vi "Add and Update Devicetype Variable in DB.vi"(8 "error in":errorcluster, 9 "Dont Set variables list":string[](array[string]), 10 "Devicetype variable\nCluster Data":string[][](array[string]), 11 "Device Name":string) -> (0 "error out":errorcluster, 3 "Devicetype \nvariable DB data":string[][](array[string]))   [LabVIEW 2020]
doc: "Thsis vi Update and Add Devicetype Variable in database by analysing Setings Cluster Data\nInput:\n1. Settins Cluster Data\n2. DeviceName\n3.Error In\n\nOutput:\n1. Devicetype Variable list\n2. Error out"
uses:
  Preset Query Enum.ctl
  source/Device Drivers/BaseDriver/BaseDriver.lvclass
panel:
  out "subarray":string[](array[string])
  out "Array":string[][](array[string])
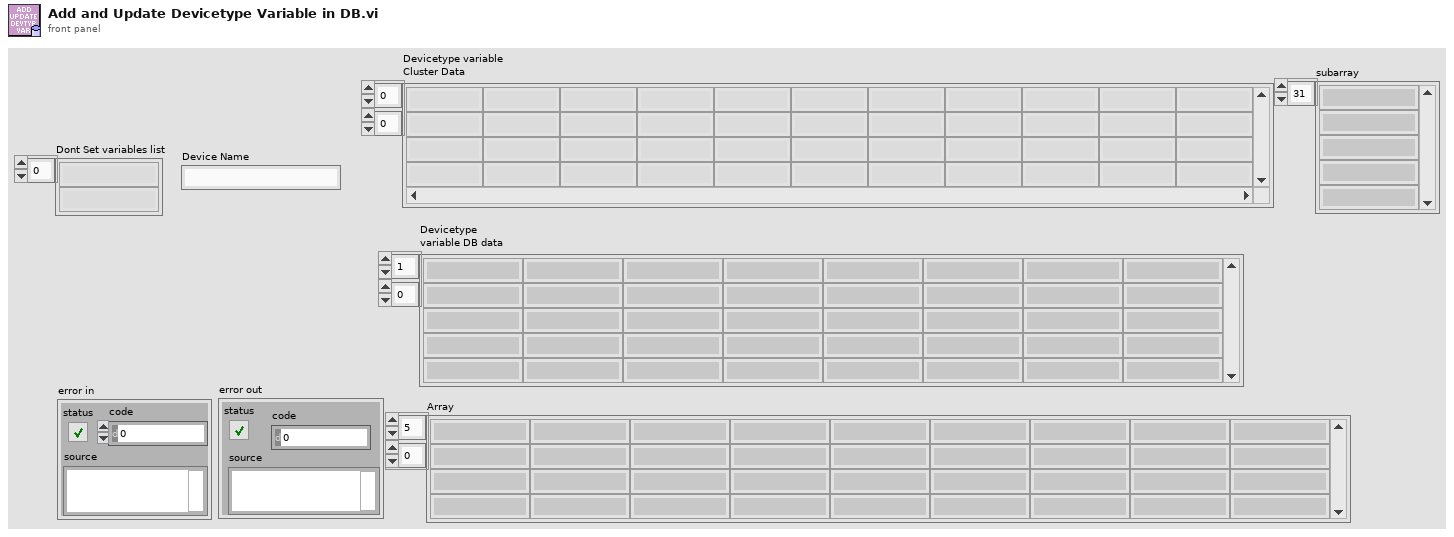
[diagram p1: front panel]
types:
  T1 = typedef "Preset Query Enum.ctl" = enum16{"Get Locations", "Get all IPs and MACs", "Get classes", "Get expt variables to set at scanstart for particular device", "Get expt devices and variables with start values", "Get expt devices and variables (with data to get)", "Get expt devices with data to get", "Get Expt devices and GUIs", "Get all devices basic properties", "Get Virtual Devices Core Info", "Get Expt names", "Get experiment basic properties", "Get experiment alarm variables", "Get MC Ports", "Get device network comm port", "Get devicetype lvclass path", "Get basic device properties", "Get Init Order", "Get all setable variables of a device", "Get device variable aliases", "Get force values of all settable variables", "Get all variables of a devicetype", "Get all variables of a device", "Get plotter details", "Get Saved Scans", "Get Scan Info", "GetGeneralGUIs", "Get expt for plotter", "Get plotter IDs from expt", "Get all devices", "Get all Virtual Devices", "Get all aliases", "Get variable and device info for Virtual Device", "GetItemLocatorIP", "Get IPs for GUIs", "Get DeviceType from Device", "GetLocalPortRange", "GetDevicePresetVariables", "Get Device Configuration", "GetAllPresetNames", "GetAllConfigurationNames", "GetPresetDeviceNames"}
  T2 = typedef "mysql_authentication.ctl" = cluster{"User":string, "Password":string, "Database":string}
  T3 = cluster{"Port":u16, "IP Address":string, "Authentication":T2}
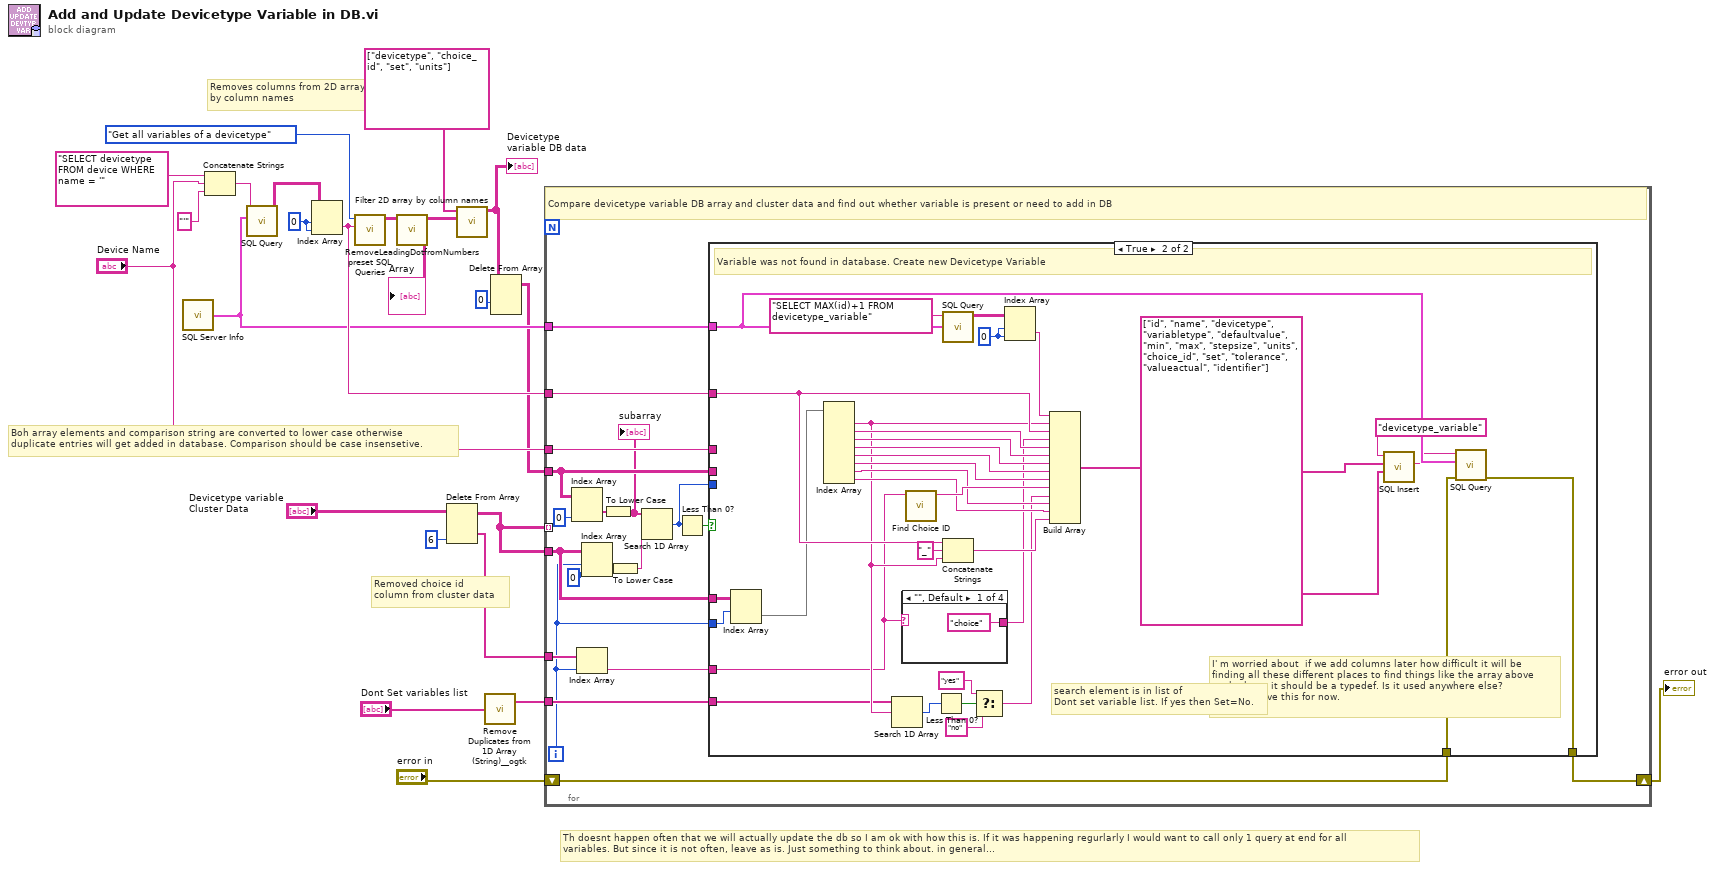
[diagram p0: block diagram]
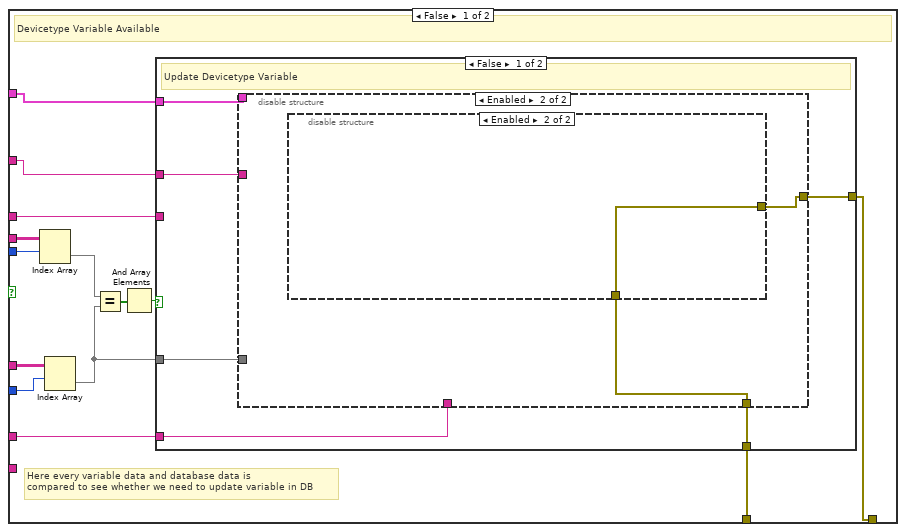
[diagram p2: hidden frame]
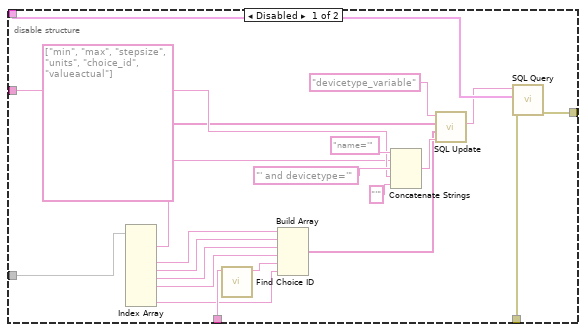
[diagram p3: hidden frame]
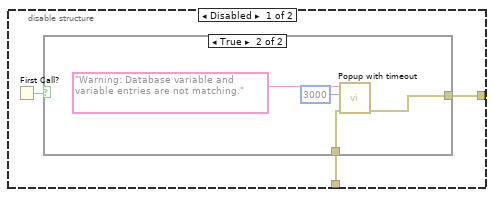
[diagram p4: hidden frame]
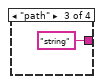
[diagram p8: hidden frame]
diagram:
  w15 = 0 ("disabled index (col)")
  # "Boh array elements and comparison string are converted to lower case otherwise \nduplicate entries will get added in database. Comparison should be case insensetive."
  # "Removed choice id\ncolumn from cluster data"
  # "Removes columns from 2D array\nby column names"
  # "Th doesnt happen often that we will actually update the db so I am ok with how this is. If it was happening regurlarly I would want to call only 1 query at end for all\nvariables. But since it is not often, leave as is. Just something to think about. in general..."
  n1 = call "SQL Server Info.vi"() -> ("SQL Server Info"=w14:T3)
  n2 = Concatenate Strings("SELECT devicetype FROM device WHERE name = '" ("Query"), "Device Name", "'" ("string")) -> (w13:string)
  n3 = call "SQL Query.vi"("SQL Server Info"=w14, "Query"=w13) -> ("data"=w16:string[][])  [unwired: 8 in, 1 out]
  n4 = Index Array(array=w16, index (row)=w15, index (col)=w15) -> (element=w20:string)
  n5 = call "preset SQL Queries.vi"("Device/Devicetype name\n/Plotter.id/ScanName#"=w20, "Preset Query"=Preset_Query_Enum."Get all variables of a devicetype") -> ("data"=w18:string[][])  [unwired: 7 in, 2 out]
  n6 = call "RemoveLeadingDotfromNumbers.vi"("data"=w18) -> ("Array"=w5:string[][])  [unwired: 10 in]
  "Array" <- w5
  n7 = Delete From Array(array="Devicetype variable\nCluster Data", index (col)=6 ("disabled index (col)")) -> (deleted portion=w22:string[], array with subset deleted=w23:string[][])  [unwired: 2 in]
  n8 = call "Filter 2D array by column names.vi"("Array in"=w5, "Array 3"=string[] ["devicetype", "choice_id", "set", "units"]) -> ("Array out"=w4:string[][])  [unwired: 9 in]
  "Devicetype \nvariable DB data" <- w4
  n9 = call "Remove Duplicates from 1D Array (String)__ogtk.vi"("Input Array"="Dont Set variables list") -> ("Output Array"=w7:string[])  [unwired: 1 out]
  n10 = Delete From Array(array=w4, index (row)=0) -> (array with subset deleted=w2:string[][])  [unwired: 2 in, 1 out]
  n11 = for {
    tunnel: w23 -> [w39]
    tunnel: w2 -> [w33]
    tunnel: w23 -> [_] mode=indexing
    tunnel: w14 -> [w38]
    tunnel: w20 -> [w34]
    shift-right: [w37] -> w9
    shift-left: "error in" -> [w36]
    tunnel: "Device Name" -> [w35]
    tunnel: w22 -> [w31]
    tunnel: w7 -> [w32]
    i -> [w30]
    # "Compare devicetype variable DB array and cluster data and find out whether variable is present or need to add in DB"
    n12 = Index Array(array=w33, index (col)=0) -> (element=w26:string[])  [unwired: 1 in]
    n13 = Index Array(array=w31, index=w30) -> (element=w29:string)
    n14 = Index Array(array=w39, index (row)=w30, index (col)=0 ("disabled index (col)")) -> (element=w27:string)
    n15 = To Lower Case(string=w26) -> (all lower case string=w25:string[])
    "subarray" <- w25
    n16 = To Lower Case(string=w27) -> (all lower case string=w24:string)
    n17 = Search 1D Array(1D array=w25, element=w24) -> (index of element=w28:i32)  [unwired: 1 in]
    n18 = Less Than 0?(x=w28) -> (x < 0?=w40:bool)
    n19 = case shown="True" w40 {
      tunnel: w33 -> [w56 _]
      tunnel: w39 -> [w55 w125]
      tunnel: w30 -> [w54 w124]
      tunnel: w38 -> [w48 w111]
      tunnel: w34 -> [w49 w116]
      tunnel: w36 -> [w47 w113]
      tunnel: [w46 w112] -> w37
      tunnel: w35 -> [w45 _]
      tunnel: w29 -> [w44 w99]
      tunnel: w32 -> [_ w106]
      tunnel: w28 -> [w43 _]
      frame False {
        # "Here every variable data and database data is \ncompared to see whether we need to update variable in DB"
        # "Devicetype Variable Available"
        n20 = Index Array(array=w56, index (row)=w43) -> (element=w52:string[])  [unwired: 1 in]
        n21 = Index Array(array=w55, index (row)=w54) -> (element=w50:string[])  [unwired: 1 in]
        n22 = Equal?(x=w52, y=w50) -> (x = y?=w53:bool[])
        n23 = And Array Elements(Boolean array=w53) -> (logical AND=w51:bool)
        n24 = case shown="False" w51 {
          tunnel: w50 -> [w60 _]
          tunnel: w49 -> [w62 _]
          tunnel: w48 -> [w61 _]
          tunnel: w47 -> [w59 w95]
          tunnel: [w58 w95] -> w46
          tunnel: w45 -> [_ _]
          tunnel: w44 -> [w57 _]
          frame False {
            # "Update Devicetype Variable"
            n25 = disable-structure shown="Enabled" {
              disable-tunnel: w62 -> [w78 _]
              disable-tunnel: w61 -> [w77 _]
              disable-tunnel: w60 -> [w74 _]
              disable-tunnel: w59 -> [w67 w85]
              disable-tunnel: [w66 w84] -> w58
              disable-tunnel: w57 -> [w65 _]
              frame Disabled {
                n26 = Index Array(array=w74) -> (element #1=w63:string, element #3=w73:string, element #4=w72:string, element #5=w71:string, element #6=w70:string, element #8=w64:string)  [unwired: 8 in, 2 out]
                n27 = call "Find Choice ID.vi"("Enum"=w65) -> ("Choice ID"=w69:string)  [unwired: 9 in, 1 out]
                n28 = Build Array(w73, w72, w71, w70, w69, w64) -> (w68:string[])
                n29 = Concatenate Strings("name='", w63, "' and devicetype='", w78, "'") -> (w79:string)
                n30 = call "SQL Update.vi"("Where clause"=w79, "Values"=w68, "Column Names"=string[] ["min", "max", "stepsize", "units", "choice_id", "valueactual"], "Table"="devicetype_variable") -> ("Query String"=w76:string)  [unwired: 7 in]
                n31 = call "SQL Query.vi"("error in (no error)"=w67, "SQL Server Info"=w77, "Query"=w76) -> ("error out"=w66:errorcluster)  [unwired: 7 in, 1 out]
              }
              frame Enabled {
                n32 = disable-structure shown="Enabled" {
                  disable-tunnel: w85 -> [w87 w94]
                  disable-tunnel: [w86 w94] -> w84
                  frame Disabled {
                    n33 = First Call?() -> (First Call?: T/F=w88:bool)
                    n34 = case shown="True" w88 {
                      tunnel: w87 -> [w89 w91]
                      tunnel: [w89 w90] -> w86
                      frame False {
                      }
                      frame True {
                        n35 = call "Popup with timeout.vi"("error"=w91, "timeout"=u32 3000, "message"="Warning: Database variable and variable entries are not matching.") -> ("error out"=w90:errorcluster)  [unwired: 8 in]
                      }
                    }
                  }
                  frame Enabled {
                  }
                }
              }
            }
          }
          frame True {
          }
        }
      }
      frame True {
        w127 = 0 ("disabled index (col)")
        # "I' m worried about  if we add columns later how difficult it will be\nfinding all these different places to find things like the array above\nat the least it should be a typedef. Is it used anywhere else?\nNo. OK. Leave this for now."
        # "search element is in list of \nDont set variable list. If yes then Set=No."
        # "Variable was not found in database. Create new Devicetype Variable"
        n36 = Index Array(array=w125, index (row)=w124) -> (element=w100:string[])  [unwired: 1 in]
        n37 = Index Array(array=w100) -> (element #1=w107:string, element #2=w122:string, element #3=w121:string, element #4=w120:string, element #5=w119:string, element #6=w118:string, element #7=w109:string, element #8=w108:string)  [unwired: 8 in]
        n38 = Search 1D Array(1D array=w106, element=w107) -> (index of element=w105:i32)  [unwired: 1 in]
        n39 = case shown="\"\", Default" w99 {
          selector: w99 -> [_ w131 _ w133]
          tunnel: ["choice" w131 "string" w133] -> w98
          frame "", Default {
          }
          frame "numeric" {
          }
          frame "path" {
          }
          frame "string" {
          }
        }
        n40 = call "Find Choice ID.vi"("Enum"=w99) -> ("Choice ID"=w117:string)  [unwired: 9 in, 1 out]
        n41 = Less Than 0?(x=w105) -> (x < 0?=w104:bool)
        n42 = call "SQL Query.vi"("SQL Server Info"=w111, "Query"="SELECT MAX(id)+1 FROM devicetype_variable") -> ("data"=w126:string[][])  [unwired: 8 in, 1 out]
        n43 = Concatenate Strings(w116, "_" ("string"), w107) -> (w110:string)
        n44 = Select(t="yes" ("element"), s=w104, f="no" ("element")) -> (s? t:f=w101:string)
        n45 = Index Array(array=w126, index (row)=w127, index (col)=w127) -> (element=w123:string)
        n46 = Build Array(w123, w107, w116, w98, w122, w121, w120, w119, w118, w117, w101, w109, w108, w110) -> (w114:string[])
        n47 = call "SQL Insert.vi"("Values"=w114, "Column Names"=string[] ["id", "name", "devicetype", "variabletype", "defaultvalue", "min", "max", "stepsize", "units", "choice_id", "set", "tolerance", "valueactual", "identifier"], "Table"="devicetype_variable") -> ("Query String"=w96:string)  [unwired: 8 in]
        n48 = call "SQL Query.vi"("error in (no error)"=w113, "SQL Server Info"=w111, "Query"=w96) -> ("error out"=w112:errorcluster)  [unwired: 7 in, 1 out]
      }
    }
  }
  "error out" <- w9
